vi "LVClass_Image ctor from HIMG file.vi"(0 "Image (const)":refnum<class "Image.lvclass">, 5 "Path to image file":path, 11 "error in (no error)":errorcluster) -> (4 "Image (new)":refnum<class "Image.lvclass">, 15 "error out":errorcluster)   [LabVIEW 2020, in "Image.lvclass"]
doc: "Image constructor from file.\n\n--------------------------------------------------------------------------------\n\n<B>ImageIn </B> : Constant Pointer to Image object.\n<B>ImageOut </B> : Constant Pointer to Image object.\n<B>image_file_path </B> : Absolute path to image file.\n<B>ErrorIn </B> : Error\n<B>ErrorOut </B> : Error\n\n--------------------------------------------------------------------------------"
uses:
  Image.lvclass
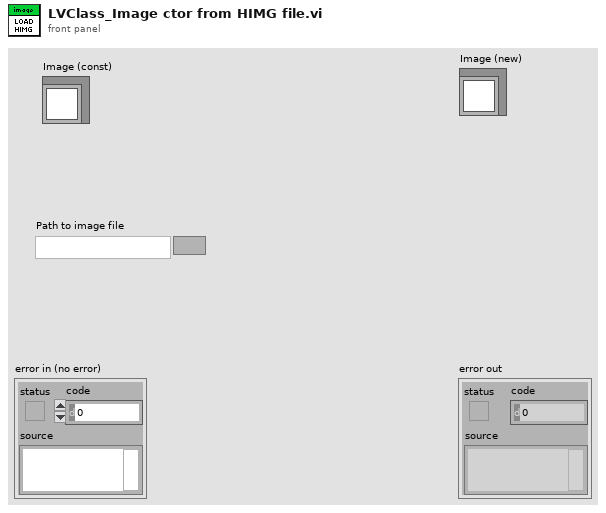
[diagram p1: front panel]
types:
  T1 = typedef "HIMG File information.ctl" = cluster{"HasoSerialNumber":string, "CameraNumber":string, "Number of bits":T2, "Size":T3, "Time Stamp":timestamp, "Number of summed images":i32, "Exposure duration spe (us)":i32, "Exposure duration real (us)":i32, "Gain":sgl}
  T2 = typedef "Data alignment enum.ctl" = enum16{"8", "16", "32"}
  T3 = typedef "Point2D.ctl" = cluster{"X":u32, "Y":u32}
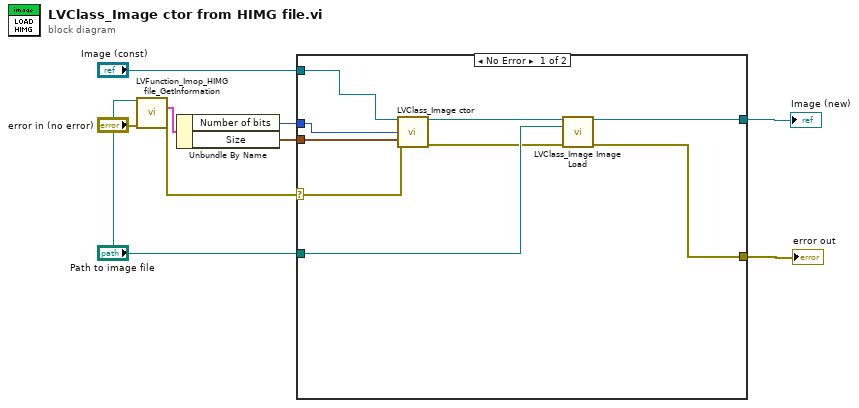
[diagram p0: block diagram]
diagram:
  n1 = call "LVFunction_Imop_HIMG file_GetInformation.vi"("Configuration file path"="Path to image file", "error in (no error)"="error in (no error)") -> ("Image info"=w6:T1, "error out"=w4:errorcluster)  [unwired: 11 in, 1 out]
  n2 = Unbundle By Name(w6) -> ("Number of bits"=w1:T2, "Size"=w7:T3)
  n3 = case shown="No Error" w4 {
    selector: w4 -> [w18 w19]
    tunnel: [w12 w19] -> w9
    tunnel: [w13 _] -> w8
    tunnel: "Path to image file" -> [w15 _]
    tunnel: w7 -> [w17 _]
    tunnel: "Image (const)" -> [w11 _]
    tunnel: w1 -> [w10 _]
    frame No Error {
      n4 = call "LVClass_Image ctor.vi"("Image (const)"=w11, "Data alignment"=w10, "Size"=w17, "error in (no error)"=w18) -> ("Image (new)"=w16:refnum<class "Image.lvclass">, "error out"=w14:errorcluster)  [unwired: 10 in]
      n5 = call "LVClass_Image Image Load.vi"("Image in"=w16, "path"=w15, "error in (no error)"=w14) -> ("Image out"=w13:refnum<class "Image.lvclass">, "error out"=w12:errorcluster)  [unwired: 11 in]
    }
    frame Error {
    }
  }
  "error out" <- w9
  "Image (new)" <- w8
